vi "WPI_CameraGet Image From Controller_Custom.vi"(4 "Camera Settings":T1={"fps"=30, "compression"=30, "Image Size"=enum."320x240", "Brightness"=30}, 5 "port":u16=1180, 6 "USB":bool, 7 "Camera Mode":u16(ring) items=["Camera Off", "USB Camera SW", "USB Camera HW", "IP Camera"], 8 "error in (no error)":errorcluster, 9 "Close?":bool, 10 "Controller Address":string, 11 "Image":T3) -> (0 "error out":errorcluster, 2 "Bandwidth (Mbps)":dbl=30.0, 3 "Image Out":T3(plugin-control))   [LabVIEW 2015]
doc: "Retrieves a specific image from the image data that the camera connected to the CompactRIO device you specify acquired. Use this VI in the FRC dashboard project on the host computer.\n\nThis software is licensed. Open the labview\\readme\\WPI Robotics Library Open Source License.txt file for more information."
uses:
  <vilib>/vision/Image Controls.llb/IMAQ Image.ctl
  <vilib>/Rock Robotics/WPI/Camera/WPI_CameraSettings Read MJPG.ctl
  <vilib>/Rock Robotics/WPI/Camera/WPI_CameraImageSize.ctl
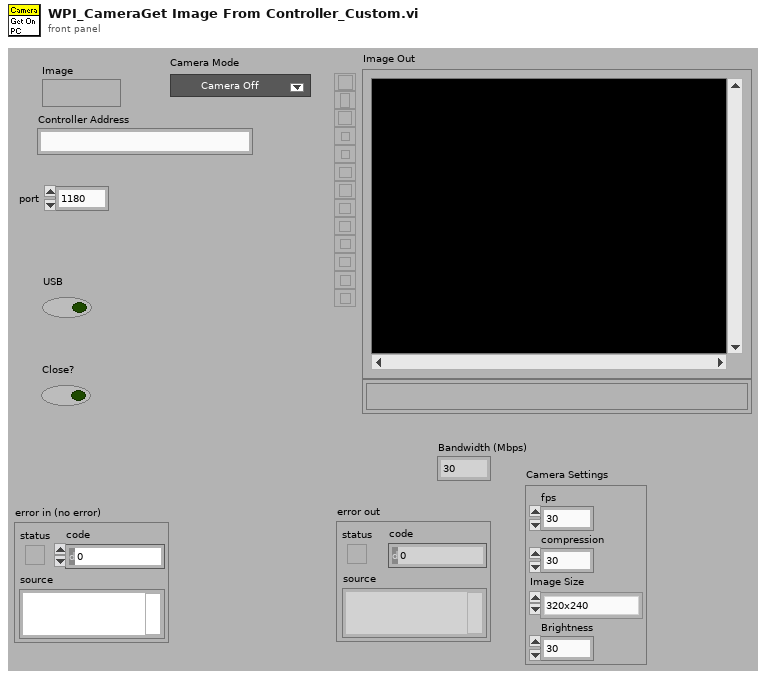
[diagram p1: front panel]
types:
  T1 = typedef "WPI_CameraSettings Read MJPG.ctl" = cluster{"fps":i32, "compression":i32, "Image Size":T2, "Brightness":i32}
  T2 = typedef "WPI_CameraImageSize.ctl" = enum16{"640x480", "320x240", "160x120", "Custom"}
  T3 = typedef "IMAQ Image.ctl" = refnum<image>
  T4 = cluster{"fps":i32, "compression":i32, i32, "Brightness":i32}
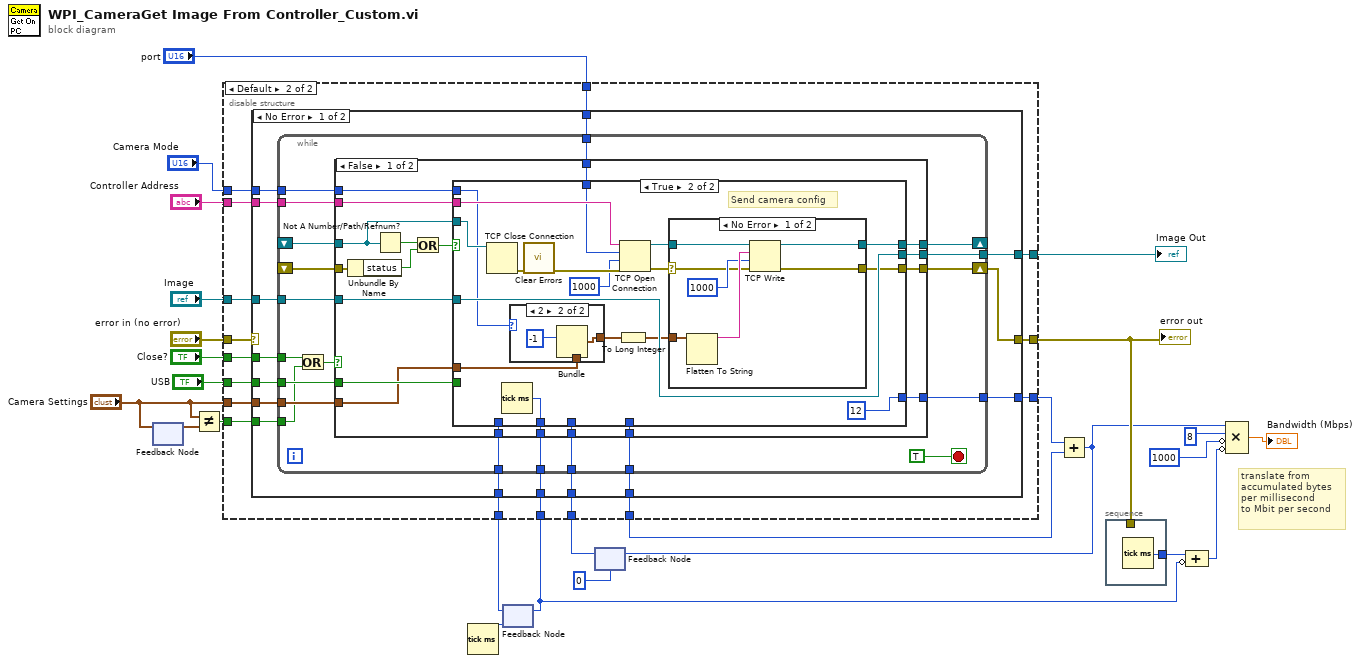
[diagram p0: block diagram]
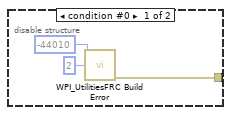
[diagram p2: hidden frame]
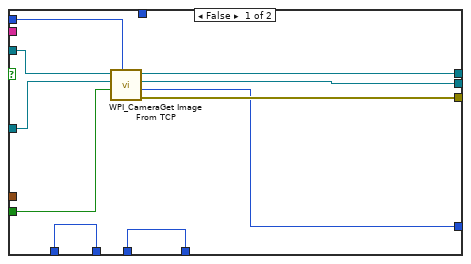
[diagram p3: hidden frame]
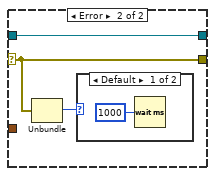
[diagram p5: hidden frame]
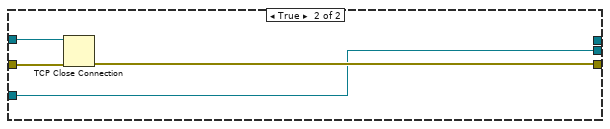
[diagram p7: hidden frame]
diagram:
  # "translate from\naccumulated bytes\nper millisecond \nto Mbit per second"
  n1 = feedback-in #1("Camera Settings") -> ()
  n2 = feedback #1() -> (w19:T1)  [unwired: 1 in]
  n3 = Not Equal?(x="Camera Settings", y=w19) -> (x != y?=w17:bool)
  n4 = Tick Count (ms)() -> (millisecond timer value=w16:u32)
  n5 = feedback #2(w16) -> (w6:u32)
  n6 = feedback #3(0) -> (w5:i32)
  n7 = disable-structure shown="Default" {
    disable-tunnel: "error in (no error)" -> [_ w44]
    disable-tunnel: [w26 w43] -> w9
    disable-tunnel: "Close?" -> [_ w42]
    disable-tunnel: "Image" -> [_ w41]
    disable-tunnel: [_ w40] -> w22
    disable-tunnel: "Controller Address" -> [_ w39]
    disable-tunnel: "USB" -> [_ w38]
    disable-tunnel: "Camera Settings" -> [_ w37]
    disable-tunnel: w17 -> [_ w36]
    disable-tunnel: [_ w35] -> w7
    disable-tunnel: w6 -> [_ w34]
    disable-tunnel: w5 -> [_ w33]
    disable-tunnel: [_ w32] -> w4
    disable-tunnel: [_ w31] -> w3
    disable-tunnel: "Camera Mode" -> [_ w30]
    disable-tunnel: "port" -> [_ w29]
    frame condition #0 {
      n8 = call <vilib>:"WPI_UtilitiesFRC Build Error.vi"("error code"=-44010 ("code"), "chain levels to remove (1)"=2) -> ("error out"=w26:errorcluster)  [unwired: 3 in, 10 out]
    }
    frame condition #1 (active) {
      n9 = case shown="No Error" w44 {
        selector: w44 -> [_ w148]
        tunnel: [w59 w148] -> w43
        tunnel: w42 -> [w58 _]
        tunnel: w41 -> [w57 w147]
        tunnel: [w56 w147] -> w40
        tunnel: w39 -> [w55 _]
        tunnel: w38 -> [w54 _]
        tunnel: w37 -> [w53 _]
        tunnel: w36 -> [w52 _]
        tunnel: [w51 w146] -> w35
        tunnel: w34 -> [w50 w146]
        tunnel: w33 -> [w49 w145]
        tunnel: [w48 w145] -> w32
        tunnel: [w47 _] -> w31
        tunnel: w30 -> [w46 _]
        tunnel: w29 -> [w45 _]
        frame No Error {
          n10 = while {
            shift-right: [w79] -> w59
            shift-left: _ -> [w77]
            shift-right: [w78] -> _
            shift-left: _ -> [w76]
            tunnel: w58 -> [w69]
            tunnel: w57 -> [w74]
            tunnel: [w73] -> w56
            tunnel: w55 -> [w72]
            tunnel: w54 -> [w71]
            tunnel: w53 -> [w70]
            tunnel: w52 -> [w67]
            tunnel: [w66] -> w51
            tunnel: w50 -> [w65]
            tunnel: w49 -> [w64]
            tunnel: [w63] -> w48
            tunnel: [w62] -> w47
            tunnel: w46 -> [w61]
            tunnel: w45 -> [w60]
            stop <- TRUE stop-if-true
            n11 = Or(x=w69, y=w67) -> (x .or. y?=w68:bool)
            n12 = case shown="False" w68 {
              tunnel: [w98 w142] -> w79
              tunnel: [w97 _] -> w78
              tunnel: w77 -> [w96 w143]
              tunnel: w76 -> [w92 w144]
              tunnel: w74 -> [w91 w141]
              tunnel: [w90 w141] -> w73
              tunnel: w72 -> [w89 _]
              tunnel: w71 -> [w88 _]
              tunnel: w70 -> [w87 _]
              tunnel: [w86 _] -> w66
              tunnel: w65 -> [w85 _]
              tunnel: w64 -> [w84 _]
              tunnel: [w83 _] -> w63
              tunnel: [w82 _] -> w62
              tunnel: w61 -> [w81 _]
              tunnel: w60 -> [w80 _]
              frame False {
                n13 = Unbundle By Name(w96) -> ("status"=w94:bool)
                n14 = Not A Number/Path/Refnum?(number/path/refnum=w92) -> (NaN/Path/Refnum?=w95:bool)
                n15 = Or(x=w95, y=w94) -> (x .or. y?=w93:bool)
                n16 = case shown="True" w93 {
                  tunnel: [w108 w116] -> w98
                  tunnel: [w106 w117] -> w97
                  tunnel: w92 -> [w107 w125]
                  tunnel: w91 -> [w105 w121]
                  tunnel: [w104 w121] -> w90
                  tunnel: w89 -> [_ w120]
                  tunnel: w88 -> [w103 _]
                  tunnel: w87 -> [_ w112]
                  tunnel: [w102 w114] -> w86
                  tunnel: w85 -> [w102 _]
                  tunnel: w84 -> [w100 _]
                  tunnel: [w100 _] -> w83
                  tunnel: [w101 12 ("timeout ms (wait forever: -1)")] -> w82
                  tunnel: w81 -> [w99 w110]
                  tunnel: w80 -> [_ w109]
                  frame False {
                    n17 = call <vilib>:"WPI_CameraGet Image From TCP.vi"("Camera Mode"=w99, "USB"=w103, "Image In"=w105, "connection ID"=w107) -> ("error out"=w108:errorcluster, "Size"=w101:i32, "Image Out"=w104:T3, "connection ID (dup)"=w106:refnum<k5>)  [unwired: 2 in, 2 out]
                  }
                  frame True {
                    # "Send camera config"
                    n18 = TCP Close Connection(connection ID=w125) -> (error out=w124:errorcluster)  [unwired: 1 in, 2 out]
                    n19 = Tick Count (ms)() -> (millisecond timer value=w114:u32)
                    n20 = case shown="2" w110 {
                      tunnel: w112 -> [w126 w129]
                      tunnel: [w126 w128] -> w111
                      frame 0, Default {
                      }
                      frame 2 {
                        n21 = Bundle(cluster=w129, "compression"=-1) -> (w128:T1)  [unwired: 3 in]
                      }
                    }
                    n22 = call <vilib>:"Clear Errors.vi"("error in (no error)"=w124) -> ("error out"=w123:errorcluster)  [unwired: 1 in, 5 out]
                    n23 = To Long Integer(number=w111) -> (32bit integer=w115:T4)
                    n24 = TCP Open Connection(address=w120, remote port or service name=w109, timeout ms (60000)=1000 ("timeout ms (wait forever: -1)"), error in (no error)=w123) -> (connection ID=w119:refnum<k5>, error out=w118:errorcluster)  [unwired: 1 out]
                    n25 = case shown="No Error" w118 {
                      selector: w118 -> [w130 w137]
                      tunnel: w119 -> [w136 w138]
                      tunnel: [w132 w138] -> w117
                      tunnel: [w131 w137] -> w116
                      tunnel: w115 -> [w135 _]
                      frame No Error {
                        n26 = Flatten To String(anything=w135) -> (data string=w134:string)  [unwired: 3 in, 2 out]
                        n27 = TCP Write(connection ID=w136, data in=w134, error in (no error)=w130, 9:1000 ("timeout ms (25000)")) -> (connection ID out=w132:refnum<k5>, error out=w131:errorcluster)  [unwired: 1 out]
                      }
                      frame Error {
                        n28 = Unbundle(w137) -> ("code"=w139:i32)  [unwired: 2 out]
                        n29 = case shown="Default" w139 {
                          frame Default {
                            n30 = Wait (ms)(milliseconds to wait=u32 1000) -> ()  [unwired: 1 out]
                          }
                          frame 56 {
                          }
                        }
                      }
                    }
                  }
                }
              }
              frame True {
                n31 = TCP Close Connection(connection ID=w144, error in (no error)=w143) -> (error out=w142:errorcluster)  [unwired: 2 out]
              }
            }
          }
        }
        frame Error {
        }
      }
    }
  }
  "error out" <- w9
  "Image Out" <- w22
  n32 = feedback-in #2(w7) -> ()
  n33 = Add(x=w3, y=w4) -> (x+y=w8:i32)
  n34 = feedback-in #3(w8) -> ()
  n35 = stacked-sequence {
    tunnel: [w149] -> w12
    tunnel: w9 -> [_]
    frame #0 {
      n36 = Tick Count (ms)() -> (millisecond timer value=w149:u32)
    }
  }
  n37 = Compound Arithmetic op=ADD(w12, invert w7) -> (w13:u32)
  n38 = Compound Arithmetic op=MULTIPLY(w8, 8 ("timeout ms (25000)"), invert 1000 ("timeout ms (25000)"), invert w13) -> (→"Bandwidth (Mbps)":dbl)
